vi "Main Queue Driver.vi"(0 "Queue Name":string, 5 "State":T1, 7 "State []":T1[](array[typedef]), 11 "error in (no error)":errorcluster, 13 "Operations":T2) -> (4 "Dequeued Element":T1, 15 "error out":errorcluster)   [LabVIEW 2021]
doc: "This Vi acts a queue driver performing queue operations such as enqueue and dequeue."
uses:
  Controls/State Cluster.ctl
  Controls/Operation.ctl
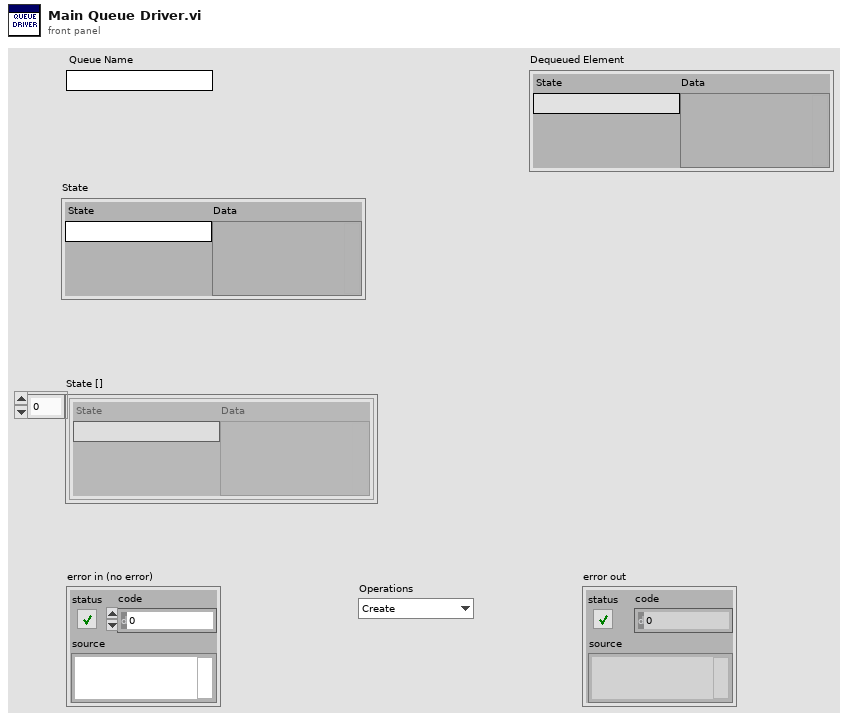
[diagram p1: front panel]
types:
  T1 = typedef "State Cluster.ctl" = cluster{"State":string, "Data":variant}
  T2 = typedef "Operation.ctl" = enum16{"Create", "Enqueue", "Enqueue N", "Enstack", "Dequeue", "Flush", "Release"}
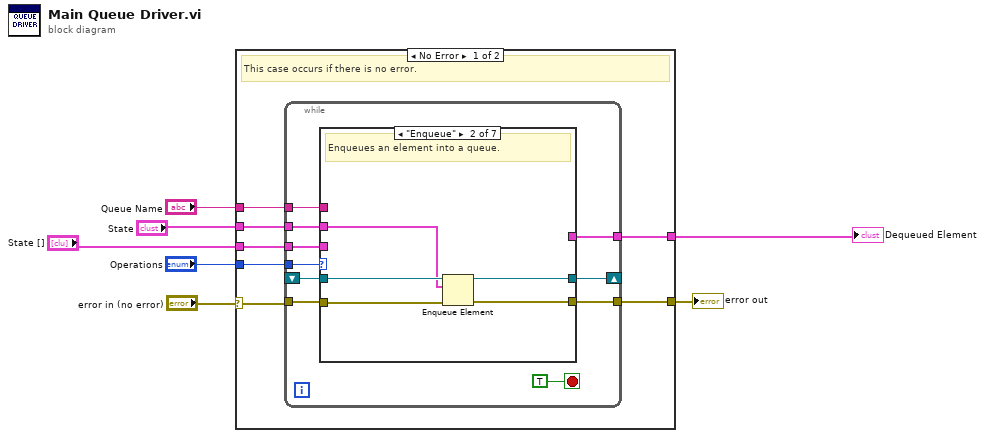
[diagram p0: block diagram]
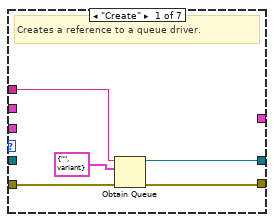
[diagram p2: hidden frame]
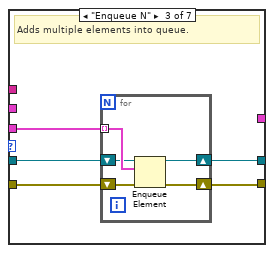
[diagram p3: hidden frame]
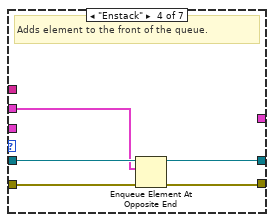
[diagram p4: hidden frame]
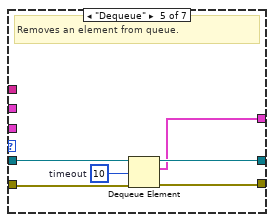
[diagram p5: hidden frame]
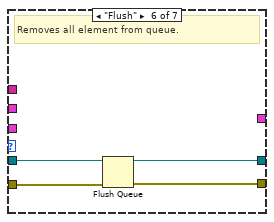
[diagram p6: hidden frame]
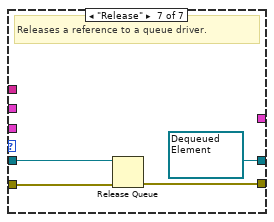
[diagram p7: hidden frame]
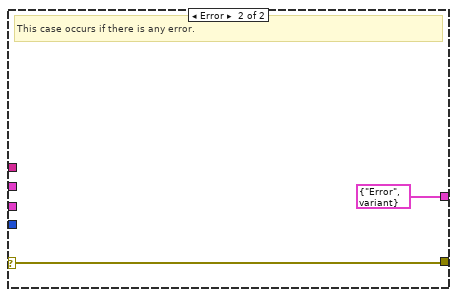
[diagram p8: hidden frame]
diagram:
  n1 = case shown="No Error" "error in (no error)" {
    selector: "error in (no error)" -> [w14 w65]
    tunnel: "Operations" -> [w13 _]
    tunnel: "State []" -> [w12 _]
    tunnel: "State" -> [w11 _]
    tunnel: "Queue Name" -> [w10 _]
    tunnel: [w9 T1 {"State"="Error", "Data"=variant} ("Dequeued Element")] -> w1
    tunnel: [w8 w65] -> w5
    frame No Error {
      # "This case occurs if there is no error."
      n2 = while {
        tunnel: w13 -> [w23]
        tunnel: w12 -> [w22]
        tunnel: w11 -> [w21]
        tunnel: w10 -> [w20]
        shift-right: [w18] -> _
        shift-left: _ -> [w17]
        tunnel: [w16] -> w9
        tunnel: w14 -> [w24]
        tunnel: [w19] -> w8
        stop <- TRUE stop-if-true
        n3 = case shown="\"Enqueue\"" w23 {
          tunnel: w24 -> [w29 w34 w39 w49 w55 w59 w63]
          tunnel: w22 -> [_ _ w37 _ _ _ _]
          tunnel: w21 -> [_ w30 _ w46 _ _ _]
          tunnel: w20 -> [w27 _ _ _ _ _ _]
          tunnel: [w28 w33 w38 w48 w54 w58 w62] -> w19
          tunnel: [w26 w31 w35 w45 w51 w56 refnum<queue> refnum ("queue out")] -> w18
          tunnel: w17 -> [_ w32 w36 w47 w53 w57 w61]
          tunnel: [_ _ _ _ w50 _ _] -> w16
          frame "Create" {
            # "Creates a reference to a queue driver."
            n4 = Obtain Queue(name (unnamed)=w27, element data type=T1 {"State"="", "Data"=variant} ("Dequeued Element"), error in (no error)=w29) -> (queue out=w26:refnum<queue>, error out=w28:errorcluster)  [unwired: 2 in, 1 out]
          }
          frame "Enqueue" {
            # "Enqueues an element into a queue."
            n5 = Enqueue Element(queue=w32, element=w30, error in (no error)=w34) -> (queue out=w31:refnum<queue>, error out=w33:errorcluster)  [unwired: 1 in, 1 out]
          }
          frame "Enqueue N" {
            # "Adds multiple elements into queue."
            n6 = for {
              shift-right: [w43] -> w38
              shift-left: w39 -> [w44]
              tunnel: w37 -> [w42] mode=indexing
              shift-right: [w40] -> w35
              shift-left: w36 -> [w41]
              n7 = Enqueue Element(queue=w41, element=w42, error in (no error)=w44) -> (queue out=w40:refnum<queue>, error out=w43:errorcluster)  [unwired: 1 in, 1 out]
            }
          }
          frame "Enstack" {
            # "Adds element to the front of the queue."
            n8 = Enqueue Element At Opposite End(queue=w47, element=w46, error in (no error)=w49) -> (queue out=w45:refnum<queue>, error out=w48:errorcluster)  [unwired: 1 in, 1 out]
          }
          frame "Dequeue" {
            w52 = 10  # timeout
            # "Removes an element from queue."
            n9 = Dequeue Element(queue=w53, timeout in ms (-1)=w52, error in (no error)=w55) -> (queue out=w51:refnum<queue>, element=w50:T1, error out=w54:errorcluster)  [unwired: 1 out]
          }
          frame "Flush" {
            # "Removes all element from queue."
            n10 = Flush Queue(queue=w57, error in (no error)=w59) -> (queue out=w56:refnum<queue>, error out=w58:errorcluster)  [unwired: 1 out]
          }
          frame "Release" {
            # "Releases a reference to a queue driver."
            n11 = Release Queue(queue=w61, error in (no error)=w63) -> (error out=w62:errorcluster)  [unwired: 1 in, 2 out]
          }
        }
      }
    }
    frame Error {
      # "This case occurs if there is any error."
    }
  }
  "error out" <- w5
  "Dequeued Element" <- w1
